vi "Test Set Column.vi"() -> ()   [LabVIEW 2020]
uses:
  <vilib>/JDP Science/JSONtext/LVClass Serializer/JSONtext LVClass Serializer.lvclass
  41c2f27f-29b4-4a13-b62c-0480280bd3b8.vi
  4be293ec-a983-47f6-a53c-e9fe45705fff.vi
  1753aa04-4026-42d7-a3d8-2b067e0806e5.vi
panel:
  out "error out":errorcluster
  out "<JSON>":string
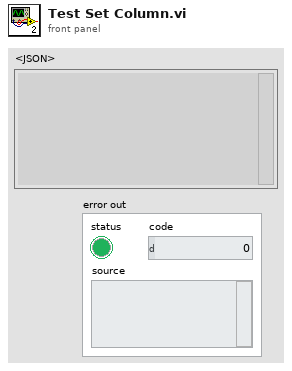
[diagram p1: front panel]
types:
  T1 = cluster{"field":string, "title":string, "Attributes":map{string, variant}}
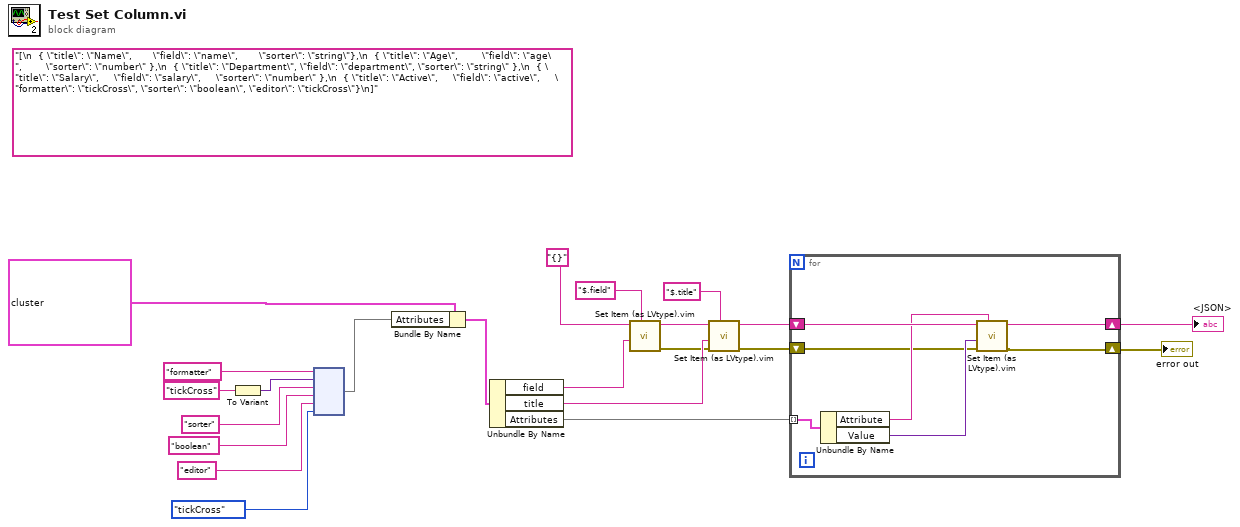
[diagram p0: block diagram]
diagram:
  (unwired) "[\n  { \"title\": \"Name\",       \"field\": \"name\",       \"sorter\": \"string\"},\n  { \"title\": \"Age\",        \"field\": \"age\",        \"sorter\": \"number\" },\n  { \"title\": \"Department\", \"field\": \"department\", \"sorter\": \"string\" },\n  { \"title\": \"Salary\",     \"field\": \"salary\",     \"sorter\": \"number\" },\n  { \"title\": \"Active\",     \"field\": \"active\",     \"formatter\": \"tickCross\", \"sorter\": \"boolean\", \"editor\": \"tickCross\"}\n]"
  n1 = To Variant(anything="tickCross" ("key")) -> (Variant=w18:variant)
  n2 = node("formatter" ("key"), w18, "sorter" ("key"), "boolean" ("key"), "editor" ("key"), enum16{"tickCross", "beanCrost", "fdsdfs"}."tickCross") -> (w21:map{string, variant})
  n3 = Bundle By Name(cluster=T1 {"field"="sdf", "title"="fvgxd", "Attributes"={}}, "Attributes"=w21) -> (w14:T1)
  n4 = Unbundle By Name(w14) -> ("field"=w10:string, "title"=w8:string, "Attributes"=w7:map{string, variant})
  n5 = call "Set Item (as LVtype).vim"("$Path or Item Name"="$.field", "Anything"=w10, "JSON"="{}") -> ("error out"=w4:errorcluster, "<JSON>"=w11:string)  [unwired: 5 in, 1 out]
  n6 = call "Set Item (as LVtype).vim"("$Path or Item Name"="$.title", "error in (no error)"=w4, "Anything"=w8, "JSON"=w11) -> ("error out"=w3:errorcluster, "<JSON>"=w6:string)  [unwired: 4 in, 1 out]
  n7 = for {
    tunnel: w7 -> [w29] mode=indexing
    shift-right: [w25] -> w5
    shift-left: w6 -> [w27]
    shift-right: [w23] -> w2
    shift-left: w3 -> [w24]
    n8 = Unbundle By Name(w29) -> ("Attribute"=w26:string, "Value"=w28:variant)
    n9 = call "Set Item (as LVtype).vim"("$Path or Item Name"=w26, "error in (no error)"=w24, "Anything"=w28, "JSON"=w27) -> ("error out"=w23:errorcluster, "<JSON>"=w25:string)  [unwired: 4 in, 1 out]
  }
  "<JSON>" <- w5
  "error out" <- w2
